vi "get file info.vi"(8 "error in":errorcluster, 11 "Video File in":refnum<class "Video File.lvclass">) -> (0 "error out":errorcluster, 3 "Video File out":refnum<class "Video File.lvclass">)   [LabVIEW 2023, in "File Classes.lvlib" / "Video File.lvclass"]
uses:
  Video File.lvclass
  D:/Library/LabVIEW Projects/Personal projects/Picture Organiser/Source Code/File Classes/File/File.lvclass
  File/File.lvclass/File.ctl
  Video File.lvclass/Video File.ctl
  File/Accessors/Read Source Path.vi
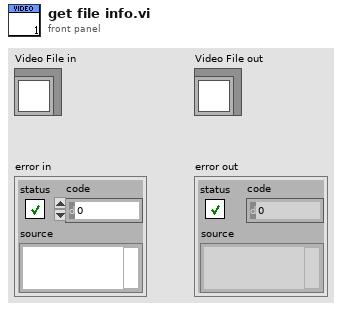
[diagram p1: front panel]
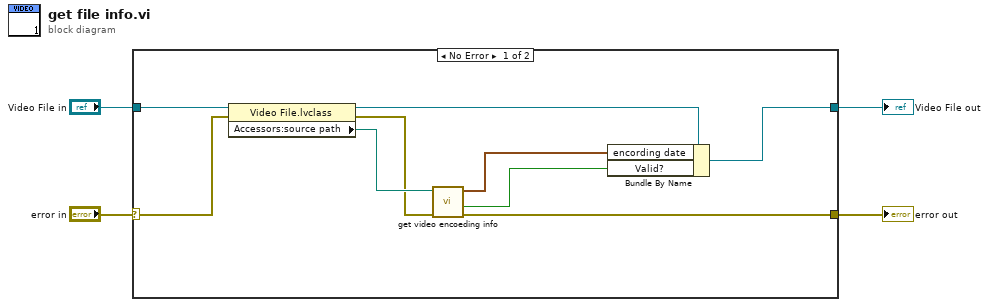
[diagram p0: block diagram]
diagram:
  n1 = case shown="No Error" "error in" {
    selector: "error in" -> [w9 w15]
    tunnel: "Video File in" -> [w5 w14]
    tunnel: [w8 w14] -> w2
    tunnel: [w7 w15] -> w1
    frame No Error {
      n2 = property class="Video File.lvclass"(reference=w5, error in=w9) -> (reference out=w6:refnum<class "Video File.lvclass">, error out=w10:errorcluster, "Accessors:source path"=w13:path)
      n3 = call "get video encoeding info.vi"("error in"=w10, "Path"=w13) -> ("error out"=w7:errorcluster, "Valid?"=w11:bool, "output 1"=w12:timestamp)  [unwired: 7 in]
      n4 = Bundle By Name(cluster=w6, "encording date"=w12, "Valid?"=w11) -> (w8:refnum<class "Video File.lvclass">)
    }
    frame Error {
    }
  }
  "error out" <- w1
  "Video File out" <- w2
